vi "Pose2DTranslate.vi"(9 "Translation Vector":T1, 11 "Starting Pose":T2) -> (3 "Resulting Pose":T2)   [LabVIEW 2018]
uses:
  Pose2D.ctl
  Vector/Vector2D.ctl
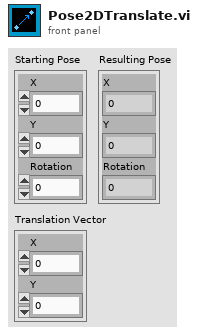
[diagram p1: front panel]
types:
  T1 = typedef "Vector2D.ctl" = cluster{"X":dbl, "Y":dbl}
  T2 = typedef "Pose2D.ctl" = cluster{"X":dbl, "Y":dbl, "Rotation":dbl}
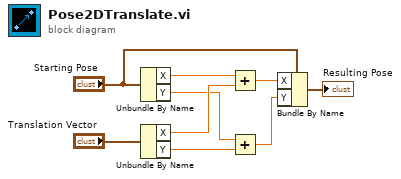
[diagram p0: block diagram]
diagram:
  n1 = Unbundle By Name("Starting Pose") -> ("X"=w8:dbl, "Y"=w5:dbl)
  n2 = Unbundle By Name("Translation Vector") -> ("X"=w7:dbl, "Y"=w6:dbl)
  n3 = Add(x=w8, y=w7) -> (x+y=w3:dbl)
  n4 = Add(x=w5, y=w6) -> (x+y=w2:dbl)
  n5 = Bundle By Name(cluster="Starting Pose", "X"=w3, "Y"=w2) -> (→"Resulting Pose":T2)
